vi "Graphics-Draw Caret (Picture).vi"(0 "picture in":picture, 7 "rect":T1, 11 "Offset":i32, 12 "color(black)":u32(colorbox)=16711680, 13 "pen":T2) -> (4 "picture out":picture)   [LabVIEW 2020]
uses:
  <vilib>/Utility/miscctls.llb/LVRectTypeDef.ctl
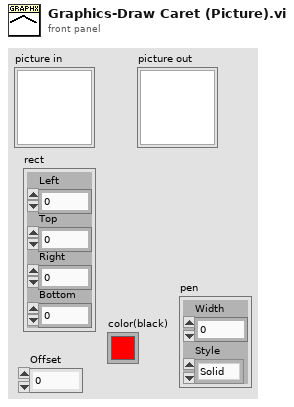
[diagram p1: front panel]
types:
  T1 = typedef "LVRectTypeDef.ctl" = cluster{"Left":i16, "Top":i16, "Right":i16, "Bottom":i16}
  T2 = cluster{"Width":u16, "Style":enum32{"Solid", "Dash", "Dot", "DashDot", "DashDotDot"}}
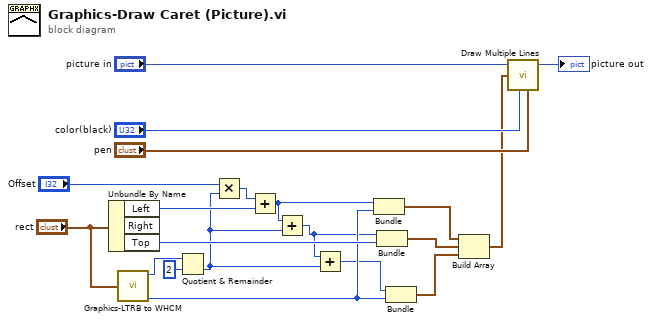
[diagram p0: block diagram]
diagram:
  n1 = Unbundle By Name("rect") -> ("Left"=w7:i16, "Top"=w16:i16)  [unwired: 1 out]
  n2 = call "Graphics-LTRB to WHCM.vi"("LTRB"="rect") -> ("Middle"=w8:i16, "Width"=w11:i16)  [unwired: 4 in, 2 out]
  n3 = Quotient & Remainder(x=w11, y=i16 2) -> (floor(x/y)=w2:i16)  [unwired: 1 out]
  n4 = Multiply(x="Offset", y=w2) -> (x*y=w4:i32)
  n5 = Add(x=w4, y=w7) -> (x+y=w5:i32)
  n6 = Add(x=w5, y=w2) -> (x+y=w3:i32)
  n7 = Add(x=w3, y=w2) -> (x+y=w1:i32)
  n8 = Bundle(w5, "Middle"=w8) -> (w12:cluster{i32, "Middle":i16})  [unwired: 1 in]
  n9 = Bundle(w3, "Top"=w16) -> (w9:cluster{i32, "Top":i16})  [unwired: 1 in]
  n10 = Bundle(w1, "Middle"=w8) -> (w14:cluster{i32, "Middle":i16})  [unwired: 1 in]
  n11 = Build Array(w12, w9, w14) -> (w13:cluster{i32, "Middle":i16}[])
  n12 = call <vilib>:"Draw Multiple Lines.vi"("picture"="picture in", "line endpoints"=w13, "color(black)"="color(black)", "pen"="pen") -> ("new picture"=→"picture out":picture)  [unwired: 5 in]
